vi "noVIPM_PostBuild.vi"() -> ()   [LabVIEW 2019]
uses:
  <vilib>/Wiresmith Technology/G CLI/Argument Parser/Option Class/Option Configuration.ctl
  <vilib>/Wiresmith Technology/G CLI/Argument Parser/Option Class/Argument Type.ctl
  VIPM/VIPM.lvlib
  <vilib>/Wiresmith Technology/G CLI/CLI Class/CLI.lvclass
  <vilib>/Wiresmith Technology/G CLI/Argument Parser/Option Set Class/Option Set.lvclass
  <vilib>/Wiresmith Technology/G CLI/Argument Parser/Option Class/Option.lvclass
panel:
  out "Post Build Custom Action File":path
  out "error out":errorcluster
  out "VIPB File":path
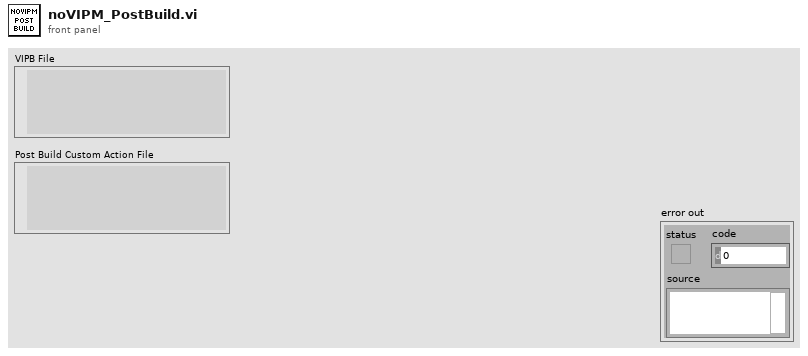
[diagram p1: front panel]
types:
  T1 = typedef "Option Parser.lvlib/Option.lvclass/Option Configuration.ctl" = cluster{"Option Type":T2, "Option Labels":string[], "Key":string, "Description":string, "Required":bool, "Default Value":string}
  T2 = typedef "Option Parser.lvlib/Option.lvclass/Argument Type.ctl" = enum16{"flag", "value"}
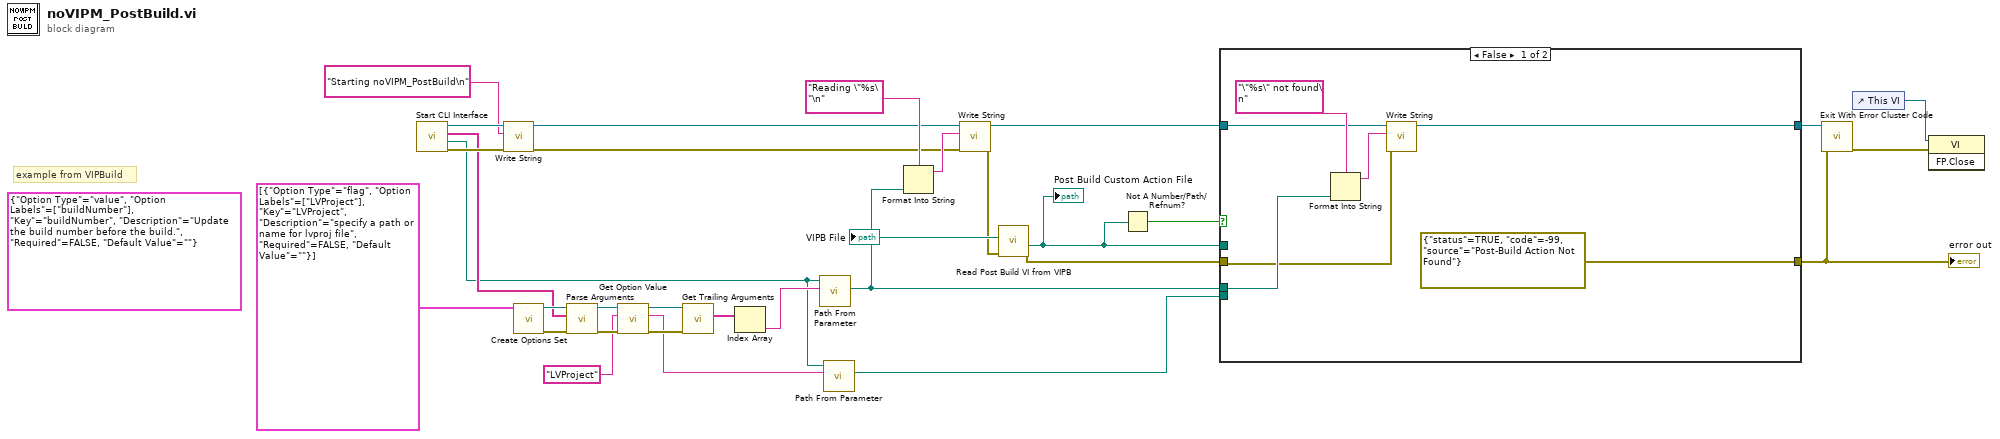
[diagram p0: block diagram]
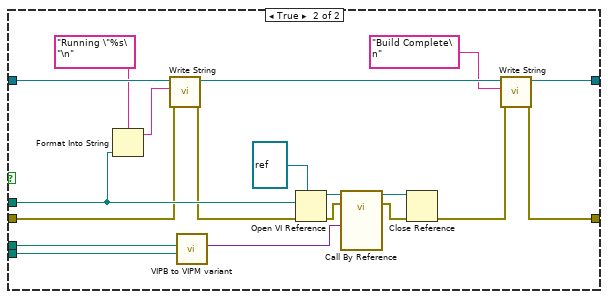
[diagram p2: hidden frame]
diagram:
  (unwired) T1 {"Option Type"=enum."value", "Option Labels"=["buildNumber"], "Key"="buildNumber", "Description"="Update the build number before the build.", "Required"=FALSE, "Default Value"=""} ("Option Config")
  # "example from VIPBuild"
  n1 = call <vilib>:"Start CLI Interface.vi"() -> ("error out"=w27:errorcluster, "Working Directory"=w1:path, "Custom Parameters"=w11:string[], "CLI out"=w29:refnum<class "CLI.lvclass">)  [unwired: 8 in]
  n2 = call <vilib>:"Write String.vi"("error in (no error)"=w27, "Text to Write"="Starting noVIPM_PostBuild\n" ("format string"), "CLI in"=w29) -> ("error out"=w18:errorcluster, "CLI out"=w21:refnum<class "CLI.lvclass">)  [unwired: 7 in]
  n3 = call <vilib>:"Create Options Set.vi"("Options"=T1[] [{"Option Type"=enum."flag", "Option Labels"=["LVProject"], "Key"="LVProject", "Description"="specify a path or name for lvproj file", "Required"=FALSE, "Default Value"=""}]) -> ("error out"=w13:errorcluster, "Option Set out"=w12:refnum<class "Option Set.lvclass">)  [unwired: 9 in]
  n4 = call <vilib>:"Parse Arguments.vi"("error in (no error)"=w13, "Arguments"=w11, "Option Set in"=w12) -> ("error out"=w6:errorcluster, "Option Set out"=w8:refnum<class "Option Set.lvclass">)  [unwired: 5 in, 2 out]
  n5 = call <vilib>:"Get Option Value.vi"("error in (no error)"=w6, "Option Key"="LVProject", "Option Set in"=w8) -> ("error out"=w5:errorcluster, "Value"=w3:string, "Option Set out"=w7:refnum<class "Option Set.lvclass">)  [unwired: 5 in, 1 out]
  n6 = call <vilib>:"Get Trailing Arguments.vi"("error in (no error)"=w5, "Option Set in"=w7) -> ("Arguments"=w10:string[])  [unwired: 7 in, 2 out]
  n7 = Index Array(array=w10) -> (element=w26:string)  [unwired: 1 in]
  n8 = call <vilib>:"Path From Parameter.vi"("Path Parameter"=w26, "Working Directory"=w1) -> ("Full Path"=w22:path)  [unwired: 9 in]
  "VIPB File" <- w22
  n9 = call <vilib>:"Path From Parameter.vi"("Path Parameter"=w3, "Working Directory"=w1) -> ("Full Path"=w2:path)  [unwired: 9 in]
  n10 = Format Into String(format string="Reading \"%s\"\n", w22) -> (resulting string=w20:string)  [unwired: 2 in, 1 out]
  n11 = call <vilib>:"Write String.vi"("error in (no error)"=w18, "Text to Write"=w20, "CLI in"=w21) -> ("error out"=w17:errorcluster, "CLI out"=w19:refnum<class "CLI.lvclass">)  [unwired: 7 in]
  n12 = call "Read Post Build VI from VIPB.vi"("error in"=w17, "VIPB File Path"=w22) -> ("error out"=w24:errorcluster, "appended path"=w15:path)  [unwired: 7 in, 1 out]
  "Post Build Custom Action File" <- w15
  n13 = Not A Number/Path/Refnum?(number/path/refnum=w15) -> (NaN/Path/Refnum?=w31:bool)
  n14 = case shown="False" w31 {
    tunnel: w22 -> [w35 w57]
    tunnel: w15 -> [_ w50]
    tunnel: w24 -> [w33 w46]
    tunnel: w19 -> [w36 w49]
    tunnel: [w34 w43] -> w25
    tunnel: [errorcluster {"status"=TRUE, "code"=-99, "source"="Post-Build Action Not Found"} ("error out") w41] -> w14
    tunnel: w2 -> [_ w39]
    frame False {
      n15 = Format Into String(format string="\"%s\" not found\n", w35) -> (resulting string=w38:string)  [unwired: 2 in, 1 out]
      n16 = call <vilib>:"Write String.vi"("error in (no error)"=w33, "Text to Write"=w38, "CLI in"=w36) -> ("CLI out"=w34:refnum<class "CLI.lvclass">)  [unwired: 7 in, 1 out]
    }
    frame True {
      n17 = Format Into String(format string="Running \"%s\"\n", w50) -> (resulting string=w51:string)  [unwired: 2 in, 1 out]
      n18 = call <vilib>:"Write String.vi"("error in (no error)"=w46, "Text to Write"=w51, "CLI in"=w49) -> ("error out"=w47:errorcluster, "CLI out"=w45:refnum<class "CLI.lvclass">)  [unwired: 7 in]
      n19 = call "VIPB to VIPM variant.vi"("LVProj"=w39, "Path to VIPB File"=w57) -> ("Variant"=w40:variant)  [unwired: 9 in]
      n20 = Open VI Reference(type specifier VI Refnum (for type only)=refnum<vi> refnum, vi path=w50, error in (no error)=w47) -> (vi reference=w56:refnum<vi>, error out=w52:errorcluster)  [unwired: 3 in]
      n21 = call-by-ref "?"(reference=w56, error in=w52, "Variant"=w40) -> (reference out=w53:refnum<vi>, error out=w54:errorcluster)  [unwired: 10 in, 1 out]
      n22 = Close Reference(reference=w53, error in (no error)=w54) -> (error out=w42:errorcluster)
      n23 = call <vilib>:"Write String.vi"("error in (no error)"=w42, "Text to Write"="Build Complete\n", "CLI in"=w45) -> ("error out"=w41:errorcluster, "CLI out"=w43:refnum<class "CLI.lvclass">)  [unwired: 7 in]
    }
  }
  "error out" <- w14
  n24 = call <vilib>:"Exit With Error Cluster Code.vi"("error in (no error)"=w14, "CLI in"=w25) -> ("error out"=w16:errorcluster)  [unwired: 9 in]
  n25 = control-ref of="This VI"() -> (w30:refnum<vi>)
  n26 = invoke class="VI" method="FP.Close"(reference=w30, error in=w16) -> ()  [unwired: 1 in, 3 out]
